vi "Process_stream.vi"(0 "VISA Refnum in":refnum<visa-resource-name>, 5 "Tare?":bool, 7 "error in (no error)":errorcluster, 11 "stop":bool) -> (12 "B xyz":dbl[][](array[numeric]), 14 "Reading":bool, 17 "Time":u32, 21 "Data Packet":string, 23 "3D Plot lvclass Array out":refnum<class "3D Plot Datatype.lvclass">[](array[class]), 24 "Sensor Output - Position (mm)":dbl[][](array[numeric]), 25 "Real dT":u32, 27 "error out":errorcluster)   [LabVIEW 2018]
uses:
  <vilib>/Math Plots/3D Math Plots/3D Plot/3D Plot Datatype/3D Plot Datatype.lvclass
  <vilib>/Utility/file.llb/Read Delimited Spreadsheet (I64).vi
  <vilib>/Math Plots/3D Math Plots/3D Surface/3D Surface Datatype/Public/Plot Helper (Matrix).vi
  <vilib>/Math Plots/3D Math Plots/3D Surface/3D Surface Datatype/3D Surface Datatype.lvclass
panel:
  in  "dT":u32=40
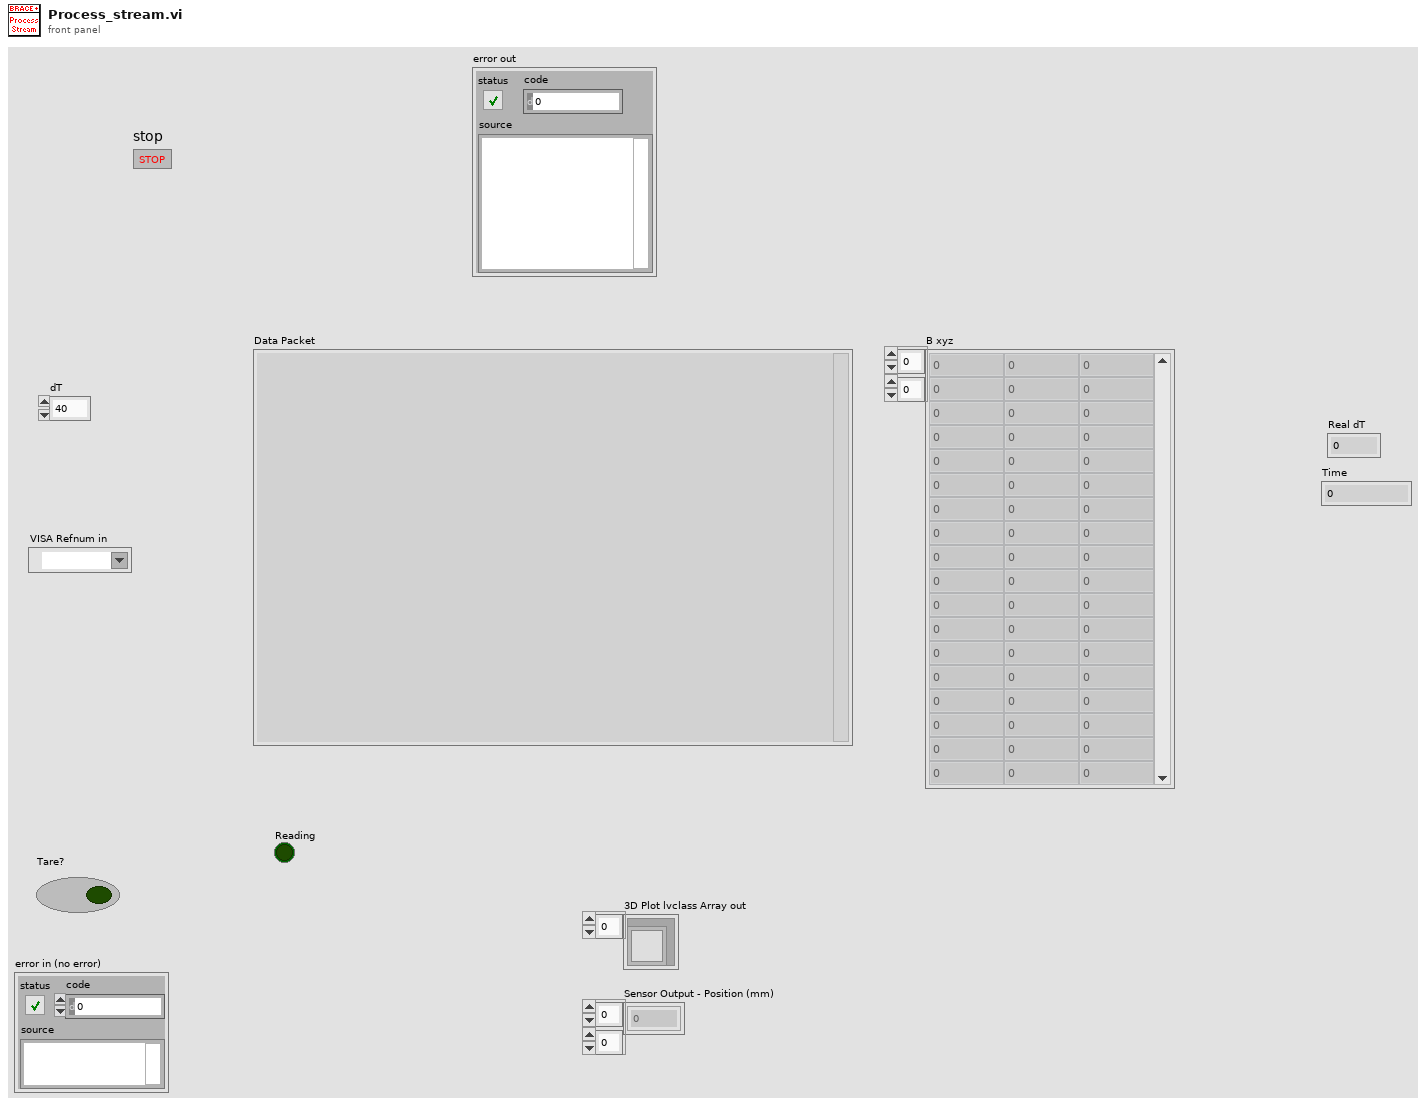
[diagram p1: front panel]
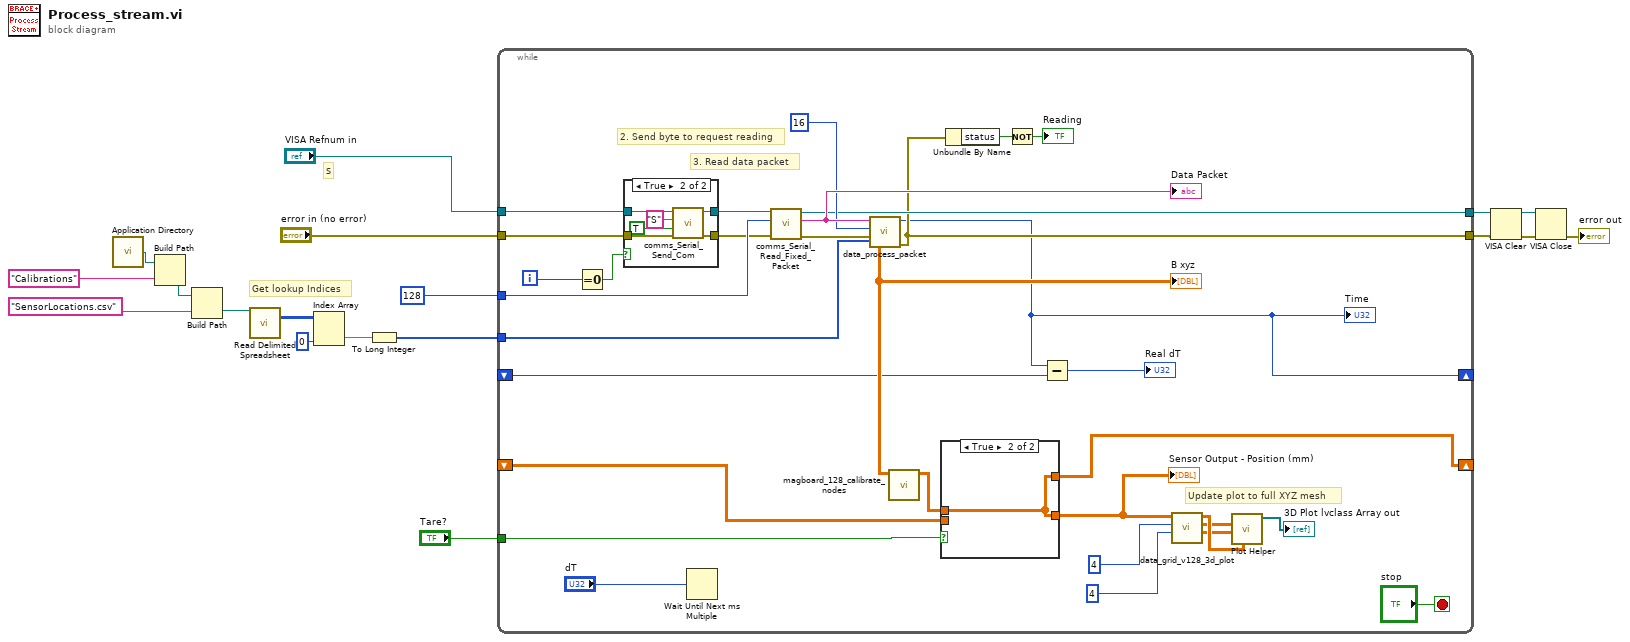
[diagram p0: block diagram]
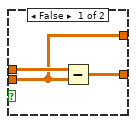
[diagram p2: hidden frame]
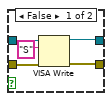
[diagram p3: hidden frame]
diagram:
  # "Get lookup Indices"
  # "S"
  n1 = call <vilib>:"Application Directory.vi"() -> ("Application Directory"=w3:path)
  n2 = Build Path(base path=w3, name or relative path="Calibrations" ("string")) -> (appended path=w5:path)
  n3 = Build Path(base path=w5, name or relative path="SensorLocations.csv" ("string")) -> (appended path=w2:path)
  n4 = call-poly <vilib>:"Read Delimited Spreadsheet.vi"("file path (dialog if empty)"=w2) -> ("all rows"=w9:i64[][])  [unwired: 9 in, 5 out]
  n5 = Index Array(array=w9, index (col)=0 ("disabled index (col)")) -> (element=w7:i64[])  [unwired: 1 in]
  n6 = To Long Integer(number=w7) -> (32bit integer=w1:i32[])
  n7 = while {
    tunnel: "Tare?" -> [w43]
    tunnel: u32 128 ("Packet Size (Bytes)") -> [w36]
    tunnel: w1 -> [w32]
    tunnel: "VISA Refnum in" -> [w29]
    shift-right: [w28] -> _
    shift-left: _ -> [w27]
    tunnel: "error in (no error)" -> [w26]
    tunnel: [w25] -> w11
    tunnel: [w24] -> w10
    shift-right: [w20] -> _
    shift-left: _ -> [w19]
    i -> [w21]
    stop <- "stop" stop-if-true
    # "Update plot to full XYZ mesh"
    # "3. Read data packet"
    # "2. Send byte to request reading"
    n8 = Equal To 0?(x=w21) -> (x = 0?=w37:bool)
    n9 = case shown="True" w37 {
      tunnel: w29 -> [w59 w65]
      tunnel: [w58 w63] -> w33
      tunnel: [w56 w62] -> w34
      tunnel: w26 -> [w55 w60]
      frame False {
        n10 = VISA Write(VISA resource name=w59, write buffer="S", error in (no error)=w55) -> (VISA resource name out=w58:refnum<visa-resource-name>, error out=w56:errorcluster)  [unwired: 1 out]
      }
      frame True {
        n11 = call "comms_Serial_Send_Com.vi"("error in"=w60, "Buffer Clear?"=TRUE, "Command"="S", "VISA resource in"=w65) -> ("error out"=w62:errorcluster, "VISA resource Out"=w63:refnum<visa-resource-name>)  [unwired: 5 in, 1 out]
      }
    }
    n12 = Wait Until Next ms Multiple(millisecond multiple="dT") -> ()  [unwired: 1 out]
    n13 = call "comms_Serial_Read_Fixed_Packet.vi"("error in"=w34, "Packet Size (Bytes)"=w36, "VISA resource in"=w33) -> ("error out"=w39:errorcluster, "Data Out"=w35:string, "VISA resource Out"=w25:refnum<visa-resource-name>)  [unwired: 4 in, 2 out]
    "Data Packet" <- w35
    n14 = call "data_process_packet.vi"("Sensor Lookup Indices"=w32, "error in (no error)"=w39, "No. Sensors"=16 ("No. Nodes"), "Binary Input Data"=w35) -> ("error out"=w24:errorcluster, "Time"=w20:u32, "Sensors (uT)"=w42:dbl[][])  [unwired: 3 in, 2 out]
    "B xyz" <- w42
    "Time" <- w20
    n15 = call "magboard_128_calibrate_nodes.vi"("Sensor Input (mT)"=w42) -> ("Sensor Output - Position (mm)"=w44:dbl[][])  [unwired: 10 in]
    n16 = case shown="True" w43 {
      tunnel: w44 -> [w53 w54]
      tunnel: w27 -> [w52 _]
      tunnel: [w52 w54] -> w28
      tunnel: [w51 w54] -> w50
      frame False {
        n17 = Subtract(x=w53, y=w52) -> (x-y=w51:dbl[][])
      }
      frame True {
      }
    }
    "Sensor Output - Position (mm)" <- w50
    n18 = Unbundle By Name(w24) -> ("status"=w40:bool)
    n19 = Not(x=w40) -> (.not. x?=→"Reading":bool)
    n20 = Subtract(x=w20, y=w19) -> (x-y=→"Real dT":u32)
    n21 = call "data_grid_v128_3d_plot.vi"("No. Rows"=4 ("Row Length"), "No. Columns"=4, "Sensor Data"=w50) -> ("Y (GRID)"=w48:dbl[][], "X (GRID)"=w47:dbl[][], "Z (GRID)"=w49:dbl[][])  [unwired: 6 in]
    n22 = call-poly <vilib>:"Plot Helper.vi"("z matrix"=w49, "y matrix"=w48, "x matrix"=w47) -> ("3D Plot lvclass Array out"=→"3D Plot lvclass Array out":refnum<class "3D Plot Datatype.lvclass">[])  [unwired: 3 in, 5 out]
  }
  n23 = VISA Clear(VISA resource name=w11, error in (no error)=w10) -> (VISA resource name out=w14:refnum<visa-resource-name>, error out=w13:errorcluster)
  n24 = VISA Close(VISA resource name=w14, error in (no error)=w13) -> (error out=→"error out":errorcluster)
